vi "Check Feedback Status.vi"(8 "error in (no error)":errorcluster, 9 "Current Set Height":dbl, 10 "Threshold (um)":dbl, 11 "Error Signal Notifier":refnum<notifier>) -> (0 "error out":errorcluster, 3 "Locked":bool)   [LabVIEW 2013, in "Automation.lvlib"]
uses:
  Automation.lvlib
  Feedback/Error Signal.ctl
  Feedback/Feedback.lvlib
panel:
  out "avg-set":dbl
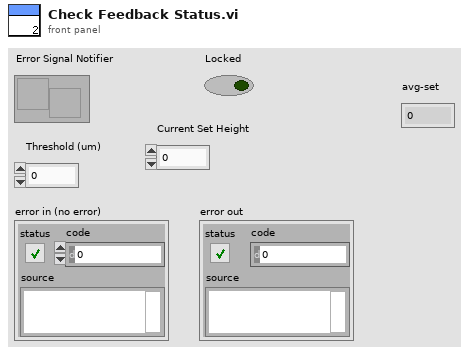
[diagram p1: front panel]
types:
  T1 = typedef "Feedback.lvlib/Error Signal.ctl" = cluster{"Error signal":dbl[], "Setpoint":dbl, "Last average":dbl}
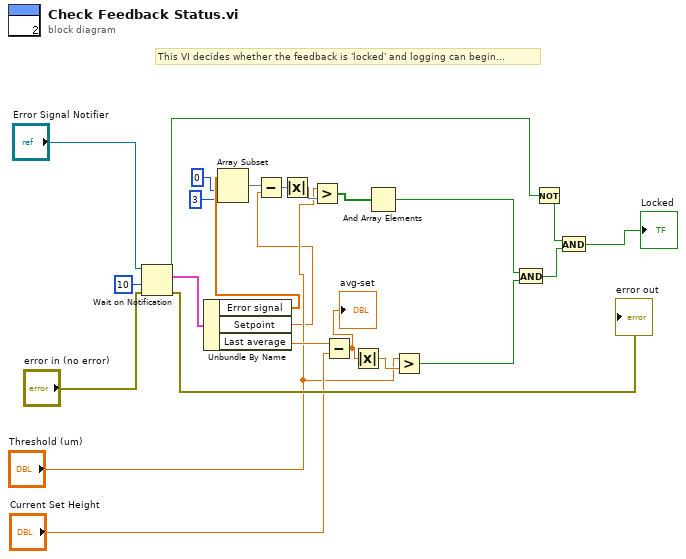
[diagram p0: block diagram]
diagram:
  # "This VI decides whether the feedback is 'locked' and logging can begin..."
  n1 = Wait on Notification(notifier="Error Signal Notifier", timeout in ms (-1)=10, error in (no error)="error in (no error)") -> (notification=w23:T1, timed out?=w9:bool, error out=→"error out":errorcluster)  [unwired: 1 in, 1 out]
  n2 = Unbundle By Name(w23) -> ("Error signal"=w19:dbl[], "Setpoint"=w5:dbl, "Last average"=w15:dbl)
  n3 = Array Subset(array=w19, index=0, length=3 ("index")) -> (w6:dbl[])
  n4 = Subtract(x=w6, y=w5) -> (x-y=w4:dbl[])
  n5 = Absolute Value(x=w4) -> (abs(x)=w12:dbl[])
  n6 = Greater?(x="Threshold (um)", y=w12) -> (0:w16:bool[])
  n7 = Subtract(x=w15, y="Current Set Height") -> (x-y=w14:dbl)
  "avg-set" <- w14
  n8 = Absolute Value(x=w14) -> (abs(x)=w11:dbl)
  n9 = And Array Elements(Boolean array=w16) -> (logical AND=w3:bool)
  n10 = Greater?(x="Threshold (um)", y=w11) -> (0:w1:bool)
  n11 = And(x=w3, y=w1) -> (x .and. y?=w2:bool)
  n12 = Not(x=w9) -> (.not. x?=w8:bool)
  n13 = And(x=w8, y=w2) -> (x .and. y?=→"Locked":bool)
